vi "Initialize_measurement.vi"() -> (2 "Graph Array":cluster{"Array":u16[], "Array":dbl[]}[](array[cluster]), 3 "Hist_array":u32[][](array[numeric]))   [LabVIEW 2019]
uses:
  Measurement_Param_Global_Var.vi
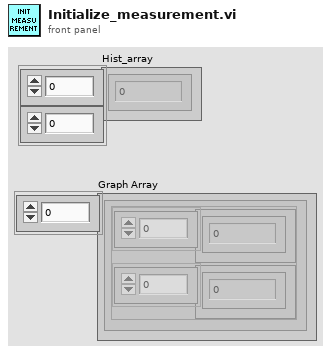
[diagram p1: front panel]
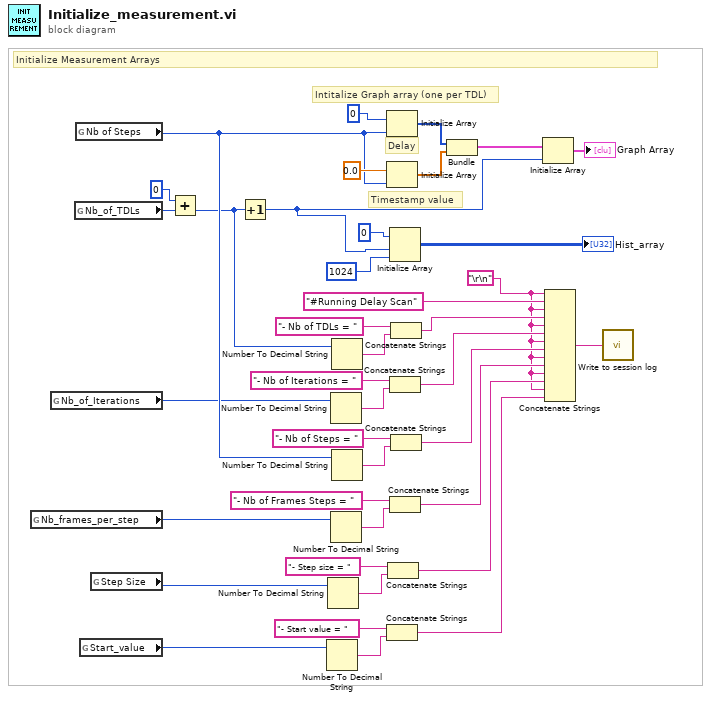
[diagram p0: block diagram]
diagram:
  w2 = "\r\n"
  # "Initialize Measurement Arrays"
  # "Timestamp value"
  # "Delay"
  # "Intitalize Graph array (one per TDL)"
  n1 = global read "Measurement_Param_Global_Var.vi" "Nb_frames_per_step"() -> (w18:u32)
  n2 = global read "Measurement_Param_Global_Var.vi" "Nb_of_Iterations"() -> (w5:u16)
  n3 = global read "Measurement_Param_Global_Var.vi" "Nb_of_TDLs"() -> (w21:u8)
  n4 = global read "Measurement_Param_Global_Var.vi" "Nb of Steps"() -> (w22:u16)
  n5 = global read "Measurement_Param_Global_Var.vi" "Start_value"() -> (w10:u16)
  n6 = global read "Measurement_Param_Global_Var.vi" "Step Size"() -> (w15:u16)
  n7 = Add(x=u8 0, y=w21) -> (x+y=w4:u8)
  n8 = Increment(x=w4) -> (x+1=w1:u8)
  n9 = Number To Decimal String(number=w10) -> (decimal integer string=w12:string)  [unwired: 1 in]
  n10 = Number To Decimal String(number=w15) -> (decimal integer string=w16:string)  [unwired: 1 in]
  n11 = Number To Decimal String(number=w5) -> (decimal integer string=w8:string)  [unwired: 1 in]
  n12 = Number To Decimal String(number=w18) -> (decimal integer string=w20:string)  [unwired: 1 in]
  n13 = Number To Decimal String(number=w4) -> (decimal integer string=w28:string)  [unwired: 1 in]
  n14 = Number To Decimal String(number=w22) -> (decimal integer string=w26:string)  [unwired: 1 in]
  n15 = Initialize Array(u16 0, w22) -> (w36:u16[])
  n16 = Initialize Array(0.0, w22) -> (w37:dbl[])
  n17 = Concatenate Strings("- Start value = " ("Session string"), w12) -> (w9:string)
  n18 = Concatenate Strings("- Step size = " ("Session string"), w16) -> (w13:string)
  n19 = Initialize Array(u32 0, w1, 1024 ("dimension size")) -> (→"Hist_array":u32[][])
  n20 = Concatenate Strings("- Nb of Iterations = " ("Session string"), w8) -> (w7:string)
  n21 = Concatenate Strings("- Nb of Frames Steps = " ("Session string"), w20) -> (w14:string)
  n22 = Concatenate Strings("- Nb of TDLs = " ("Session string"), w28) -> (w27:string)
  n23 = Concatenate Strings("- Nb of Steps = " ("Session string"), w26) -> (w24:string)
  n24 = Bundle(w36, w37) -> (w38:cluster{u16[], dbl[]})  [unwired: 1 in]
  n25 = Initialize Array(w38, w1) -> (→"Graph Array":cluster{u16[], dbl[]}[])
  n26 = Concatenate Strings(w2, "#Running Delay Scan" ("Session string"), w2, w27, w2, w7, w2, w24, w2, w14, w2, w13, w2, w9) -> (w23:string)
  n27 = call "Write to session log.vi"("Session string"=w23) -> ()  [unwired: 1 in]
